vi "Set Sender.vi"(10 "Sender":refnum<class "Sender.lvclass">, 11 "Last Ack Created Msg Strategy in":refnum<class "Last Ack Created Msg Strategy.lvclass">) -> (3 "Last Ack Created Msg Strategy out":refnum<class "Last Ack Created Msg Strategy.lvclass">)   [LabVIEW 2021, in "jettl.lvlib" / "Last Ack Created Msg Strategy.lvlib" / "Last Ack Created Msg Strategy.lvclass"]
uses:
  Last Ack Created Msg Strategy.lvclass
  Last Ack Created Msg Strategy.lvclass/Last Ack Created Msg Strategy.ctl
  Sender/Sender/Sender.lvclass
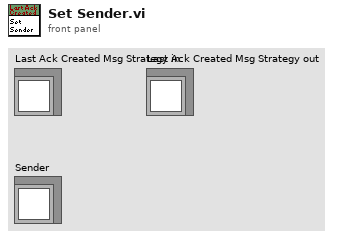
[diagram p1: front panel]
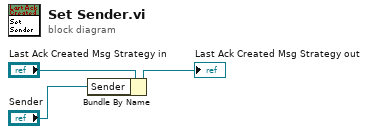
[diagram p0: block diagram]
diagram:
  n1 = Bundle By Name(cluster="Last Ack Created Msg Strategy in", "Sender"="Sender") -> (→"Last Ack Created Msg Strategy out":refnum<class "Last Ack Created Msg Strategy.lvclass">)
